vi "calculate change position.vi"(6 "parameters":T1={"max velocity (m/s)"=2.0, "wheel base width (m)"=0.7, "traverse CoF"=0.14}, 7 "Ætime (s)":dbl=0.1, 8 "initial direction":dbl, 9 "% turn":dbl(slide) scale=-100.0..100.0, 10 "m/s":dbl(slide) scale=-2.0..2.0, 11 "m/s/s":dbl(slide) scale=-1.0..1.0) -> (1 "Æ point":cluster{dbl, dbl}, 2 "end velocity (m/s)":dbl)   [LabVIEW 2009]
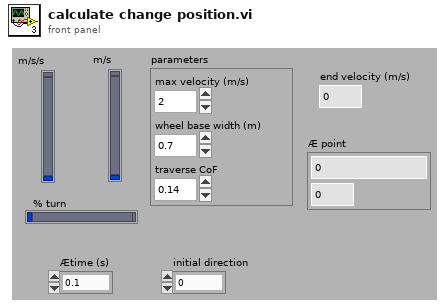
[diagram p1: front panel]
types:
  T1 = cluster{"max velocity (m/s)":dbl, "wheel base width (m)":dbl, "traverse CoF":dbl}
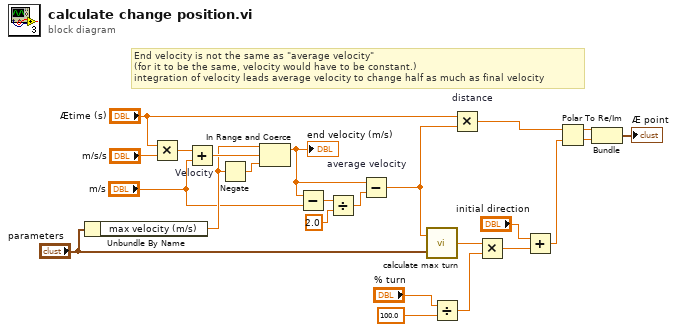
[diagram p0: block diagram]
diagram:
  # "End velocity is not the same as \"average velocity\"\n(for it to be the same, velocity would have to be constant.)\nintegration of velocity leads average velocity to change half as much as final velocity"
  n1 = Unbundle By Name("parameters") -> ("max velocity (m/s)"=w8:dbl)
  n2 = Multiply(x="Ætime (s)", y="m/s/s") -> (x*y=w21:dbl)
  n3 = Add "Velocity"(x=w21, y="m/s") -> (x+y=w10:dbl)
  n4 = Negate(x=w8) -> (-x=w7:dbl)
  n5 = In Range and Coerce(upper limit=w8, x=w10, lower limit=w7) -> (coerced(x)=w2:dbl)  [unwired: 1 out]
  "end velocity (m/s)" <- w2
  n6 = Subtract(x=w2, y="m/s") -> (x-y=w5:dbl)
  n7 = Divide(x=w5, y=2.0) -> (x/y=w3:dbl)
  n8 = Subtract "average velocity"(x=w2, y=w3) -> (x-y=w1:dbl)
  n9 = call "calculate max turn.vi"("parameters"="parameters", "Velocity (m/s)"=w1) -> ("max Ư"=w18:dbl)
  n10 = Divide(x="% turn", y=100.0) -> (x/y=w19:dbl)
  n11 = Multiply "distance"(x="Ætime (s)", y=w1) -> (x*y=w14:dbl)
  n12 = Multiply(x=w18, y=w19) -> (x*y=w16:dbl)
  n13 = Add(x="initial direction", y=w16) -> (x+y=w15:dbl)
  n14 = Polar To Re/Im(2:w15, 3:w14) -> (0:w12:dbl, 1:w13:dbl)
  n15 = Bundle(w13, w12) -> (→"Æ point":cluster{dbl, dbl})  [unwired: 1 in]
